vi "XYZStage-Verify position.vi"(8 "error in (no error)":errorcluster, 10 "XYZ Stage data":T1={"Command"=enum."Dequeue", "Channel"="Z", "X"=0.0, "Y"=0.0, "Z"=0.0, "Speed"=0, "Zero"=FALSE, "Use acknowledgement?"=TRUE} {"Speed" format="Speed= %.0f"; "Z" format="Z= %#_g"; "Y" format="Y= %#_g"; "X" format="X= %#_g"}, 11 "XYZ Stage Port":refnum<visa-resource-name>) -> (0 "error out":errorcluster)   [LabVIEW 2013]
uses:
  Typedefs/XYZ stage data.ctl
  Typedefs/XYZ stage states.ctl
  Typedefs/XYZ channel ring.ctl
  Typedefs/Command acknowledgment states.ctl
  User Interface/Windows/Position control window/Globals/Pos ctrl window globals.vi
  Global Variables/gl_UI Ctrl Refs.vi
  Globals/gl_XYZStage globals.vi
panel:
  out "Iterations":i32
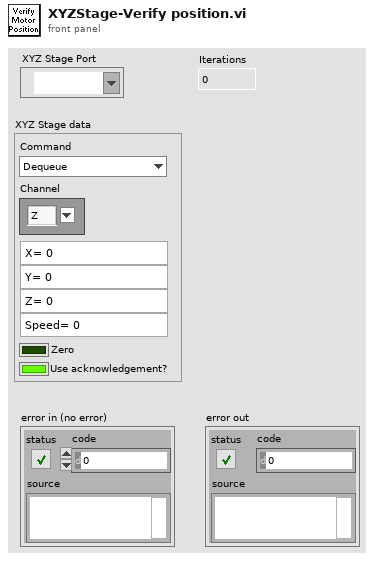
[diagram p1: front panel]
types:
  T1 = typedef "XYZ stage data.ctl" = cluster{"Command":T2, "Channel":T3, "X":sgl, "Y":sgl, "Z":sgl, "Speed":i32, "Zero":bool, "Use acknowledgement?":bool}
  T2 = typedef "XYZ stage states.ctl" = enum16{"Dequeue", "Initialize", "Read Position", "Read Speed Setting", "Move", "Set Max Speed", "Reset Axis", "Stop all movement"}
  T3 = typedef "XYZ channel ring.ctl" = string
  T4 = typedef "Command acknowledgment states.ctl" = enum16{"Acknowledge", "Wait for acknowledgment", "Release queue"}
  T5 = typedef "UI ctrl refs cluster.ctl" = cluster{"Top level VI path":path, "Top level VI ref":refnum<vi>, "User menu ref":refnum<k9>, "Sub Panel control":refnum<vi>, "Imaging Param Tab":refnum<vi>, "Occurrence-Start drivers":refnum<k4>, "Occurrence-Speed logging initialised":refnum<k4>, "Occurrence-XYZ stage initialised":refnum<k4>, "Exit button":refnum<vi>, "Status ind":refnum<vi>, "Return to Origin":refnum<vi>, "Speed Logging":refnum<vi>, "Time Lapse":refnum<vi>, "Live Imaging":refnum<vi>, "AOL Z Stack":refnum<vi>, "Motor Z Stack":refnum<vi>, "Funct Acq button":refnum<vi>, "Hard Shutter":refnum<vi>, "Virtual Shutter":refnum<vi>, "Laser Power":refnum<vi>, "AOL Mode":refnum<vi>, "Frame Size":refnum<vi>, "Field of View":refnum<vi>, "Dwell Time":refnum<vi>, "Zoom":refnum<vi>, "AOL Z":refnum<vi>, "Objective":refnum<vi>, "Axis":refnum<vi>, "Paths & Names":refnum<vi>, "Experiment folder path (ind.)":refnum<vi>, "Last State (Ind.)":refnum<vi>, "Laser wavelength ind (nm)":refnum<vi>, "Averages":refnum<vi>, "Angle (degrees)":refnum<vi>, "X centre":refnum<vi>, "Y centre":refnum<vi>, "Plane Mode":refnum<vi>, "# Planes":refnum<vi>, "Z Start":refnum<vi>, "Z Stop":refnum<vi>, "Z Step":refnum<vi>, "PMT 1":refnum<vi>, "PMT 2":refnum<vi>, "Stage XYZ Position":refnum<vi>, "Pockels@Z Start":refnum<vi>, "Pockels@Z Stop":refnum<vi>, "Obtain Z Start":refnum<vi>, "Obtain Z Stop":refnum<vi>, "Live stim.trig.period":refnum<vi>, "Live stim.trig.enable":refnum<vi>, "Funct. Acq. Pockels Modulation":refnum<vi>, "Enable Video Recording":refnum<vi>, "Video Record-Live Imaging":refnum<vi>, "Video Record-Funct acq":refnum<vi>, "AOL Z-stack Chirps Ready (ind)":refnum<vi>, "Center freq ind (nm)":refnum<vi>, "Logging queue (ind)":refnum<vi>, "Back aperture power (ind.)":refnum<vi>, "Power after objective (ind.)":refnum<vi>, "Switch user":refnum<vi>}
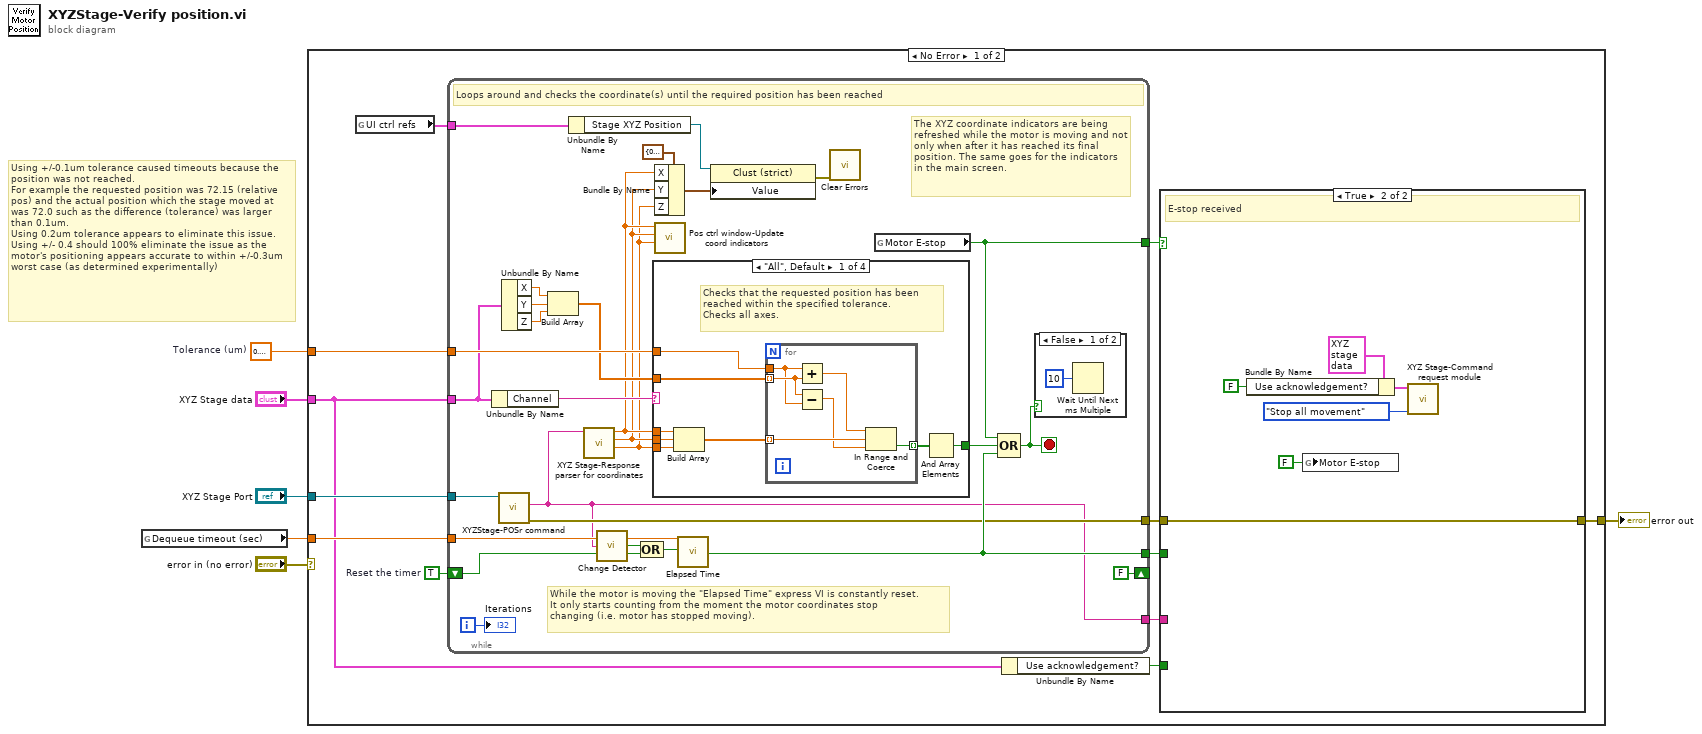
[diagram p0: block diagram]
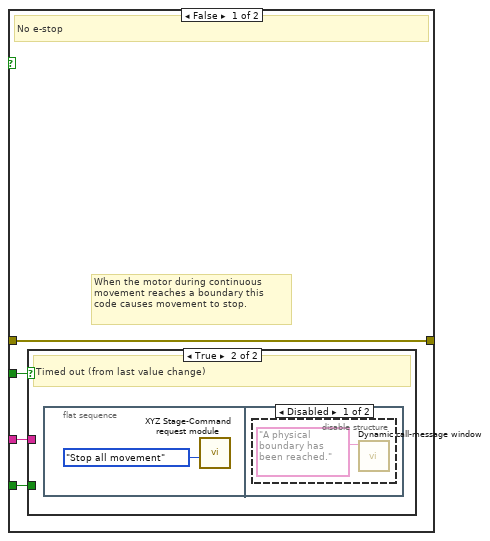
[diagram p2: hidden frame]
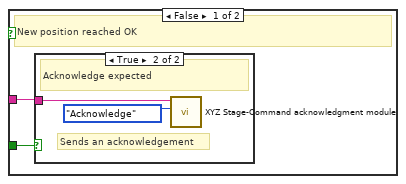
[diagram p3: hidden frame]
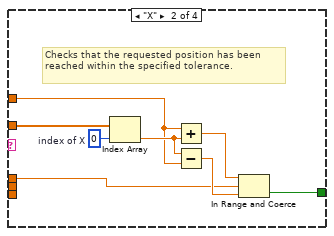
[diagram p6: hidden frame]
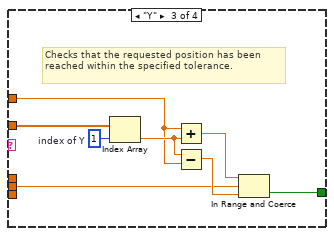
[diagram p7: hidden frame]
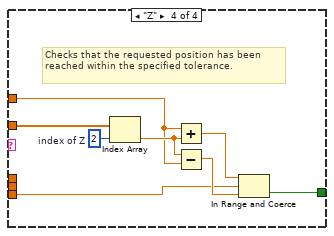
[diagram p8: hidden frame]
diagram:
  w2 = sgl 0.4  # Tolerance (um)
  # "Using +/-0.1um tolerance caused timeouts because the position was not reached.\nFor example the requested position was 72.15 (relative pos) and the actual position which the stage moved at was 72.0 such as the difference (tolerance) was larger than 0.1um.\nUsing 0.2um tolerance appears to eliminate this issue.\nUsing +/- 0.4 should 100% eliminate the issue as the motor's positioning appears accurate to within +/-0.3um worst case (as determined experimentally)"
  n1 = global read "Pos ctrl window globals.vi" "Dequeue timeout (sec)"() -> (w1:dbl)
  n2 = case shown="No Error" "error in (no error)" {
    selector: "error in (no error)" -> [_ w102]
    tunnel: "XYZ Stage data" -> [w11 _]
    tunnel: "XYZ Stage Port" -> [w18 _]
    tunnel: [w7 w102] -> w3
    tunnel: w1 -> [w16 _]
    tunnel: w2 -> [w15 _]
    frame No Error {
      w17 = TRUE  # Reset the timer
      n3 = global read "gl_UI Ctrl Refs.vi" "UI ctrl refs"() -> (w14:T5)
      n4 = while {
        tunnel: [w37] -> w8
        tunnel: w18 -> [w38]
        tunnel: w11 -> [w51]
        shift-right: [FALSE ("Send command")] -> _
        shift-left: w17 -> [w53]
        tunnel: w15 -> [w60]
        tunnel: w16 -> [w59]
        tunnel: [w56] -> w13
        tunnel: [w36] -> w12
        tunnel: w14 -> [w42]
        tunnel: [w35] -> w9
        i -> [w55]
        stop <- w58 stop-if-true
        # "The XYZ coordinate indicators are being refreshed while the motor is moving and not only when after it has reached its final position. The same goes for the indicators in the main screen."
        # "While the motor is moving the \"Elapsed Time\" express VI is constantly reset.\nIt only starts counting from the moment the motor coordinates stop \nchanging (i.e. motor has stopped moving)."
        # "Loops around and checks the coordinate(s) until the required position has been reached"
        n5 = Unbundle By Name(w51) -> ("Channel"=w61:T3)
        n6 = call "XYZStage-POSr command.vi"("VISA Refnum in"=w38) -> ("Error out"=w37:errorcluster, "read string"=w36:string)  [unwired: 7 in, 2 out]
        n7 = Unbundle By Name(w51) -> ("X"=w49:sgl, "Y"=w50:sgl, "Z"=w48:sgl)
        n8 = Build Array(w49, w50, w48) -> (w47:sgl[])
        n9 = Unbundle By Name(w42) -> ("Stage XYZ Position"=w46:refnum<vi>)
        n10 = call "XYZ Stage-Response parser for coordinates.vi"("Filtered response string (no CR)"=w36) -> ("Z"=w39:sgl, "Y"=w40:sgl, "X"=w41:sgl)  [unwired: 8 in]
        n11 = call "Change Detector.vi"("Value"=w36) -> ("Changed?"=w54:bool)
        n12 = Compound Arithmetic op=OR(w54, w53) -> (w52:bool)
        n13 = case shown="\"All\", Default" w61 {
          tunnel: w41 -> [w70 w78 _ _]
          tunnel: w40 -> [w69 _ w85 _]
          tunnel: w39 -> [w68 _ _ w93]
          tunnel: [w65 w77 w86 w94] -> w57
          tunnel: w47 -> [w64 w81 w89 w97]
          tunnel: w60 -> [w63 w79 w87 w95]
          frame "All", Default {
            # "Checks that the requested position has been reached within the specified tolerance.\nChecks all axes."
            n14 = Build Array(w70, w69, w68) -> (w67:sgl[])
            n15 = for {
              tunnel: w64 -> [w75] mode=indexing
              tunnel: w67 -> [w76] mode=indexing
              tunnel: [w72] -> w66 mode=indexing
              tunnel: w63 -> [w71]
              n16 = Add(x=w71, y=w75) -> (x+y=w74:sgl)
              n17 = Subtract(x=w75, y=w71) -> (x-y=w73:sgl)
              n18 = In Range and Coerce(upper limit=w74, x=w76, lower limit=w73) -> (In Range?=w72:bool)  [unwired: 1 out]
            }
            n19 = And Array Elements(Boolean array=w66) -> (logical AND=w65:bool)
          }
          frame "X" {
            w82 = 0  # index of X
            # "Checks that the requested position has been reached within the specified tolerance."
            n20 = Index Array(array=w81, index=w82) -> (element=w80:sgl)
            n21 = Add(x=w79, y=w80) -> (x+y=w84:sgl)
            n22 = Subtract(x=w80, y=w79) -> (x-y=w83:sgl)
            n23 = In Range and Coerce(upper limit=w84, x=w78, lower limit=w83) -> (In Range?=w77:bool)  [unwired: 1 out]
          }
          frame "Y" {
            w90 = 1  # index of Y
            # "Checks that the requested position has been reached within the specified tolerance."
            n24 = Index Array(array=w89, index=w90) -> (element=w88:sgl)
            n25 = Add(x=w87, y=w88) -> (x+y=w92:sgl)
            n26 = Subtract(x=w88, y=w87) -> (x-y=w91:sgl)
            n27 = In Range and Coerce(upper limit=w92, x=w85, lower limit=w91) -> (In Range?=w86:bool)  [unwired: 1 out]
          }
          frame "Z" {
            w98 = 2  # index of Z
            # "Checks that the requested position has been reached within the specified tolerance."
            n28 = Index Array(array=w97, index=w98) -> (element=w96:sgl)
            n29 = Add(x=w95, y=w96) -> (x+y=w100:sgl)
            n30 = Subtract(x=w96, y=w95) -> (x-y=w99:sgl)
            n31 = In Range and Coerce(upper limit=w100, x=w93, lower limit=w99) -> (In Range?=w94:bool)  [unwired: 1 out]
          }
        }
        n32 = Bundle By Name(cluster=cluster{"X":sgl, "Y":sgl, "Z":sgl} {"X"=0.0, "Y"=0.0, "Z"=0.0} ("Stage XYZ Position"), "X"=w41, "Y"=w40, "Z"=w39) -> (w44:cluster{"X":sgl, "Y":sgl, "Z":sgl})
        n33 = call "Pos ctrl window-Update coord indicators.vi"("Z"=w39, "Y"=w40, "X"=w41) -> ()  [unwired: 9 in]
        n34 = call "Elapsed Time"("Time Target (s)"=w59, "Reset"=w52) -> ("Time has Elapsed"=w56:bool)  [unwired: 10 in, 7 out]
        n35 = property on="Property Node" class="Clust (strict)"(reference=w46, "Value"=w44) -> (error out=w45:errorcluster)  [unwired: 1 in, 1 out]
        n36 = call <vilib>:"Clear Errors.vi"("error in (no error)"=w45) -> ()  [unwired: 6 in, 1 out]
        n37 = global read "gl_XYZStage globals.vi" "Motor E-stop"() -> (w35:bool)
        n38 = Compound Arithmetic op=OR(w35, w57, w56) -> (w58:bool)
        n39 = case shown="False" w58 {
          frame False {
            n40 = Wait Until Next ms Multiple(millisecond multiple=u32 10) -> ()  [unwired: 1 out]
          }
          frame True {
            # "No wait if position reached"
          }
        }
        "Iterations" <- w55
      }
      n41 = Unbundle By Name(w11) -> ("Use acknowledgement?"=w10:bool)
      n42 = case shown="True" w9 {
        tunnel: w13 -> [w22 _]
        tunnel: w12 -> [w21 _]
        tunnel: w10 -> [w20 _]
        tunnel: w8 -> [w19 w32]
        tunnel: [w19 w32] -> w7
        frame False {
          # "When the motor during continuous movement reaches a boundary this code causes movement to stop."
          # "No e-stop"
          n43 = case shown="True" w22 {
            tunnel: w21 -> [w24 _]
            tunnel: w20 -> [w23 _]
            frame False {
              # "New position reached OK"
              n44 = case shown="True" w23 {
                tunnel: w24 -> [_ w25]
                frame False {
                  # "No acknowledgement expected"
                }
                frame True {
                  # "Sends an acknowledgement"
                  # "Acknowledge expected"
                  n45 = call "XYZ Stage-Command acknowledgment module.vi"("State"=Command_acknowledgment_states."Acknowledge", "Acknowledgement Message in"=w25) -> ()  [unwired: 7 in, 3 out]
                }
              }
            }
            frame True {
              # "Timed out (from last value change)"
              n46 = flat-sequence {
                frame #0 {
                  n47 = call "XYZ Stage-Command request module.vi"("Command"=XYZ_stage_states."Stop all movement") -> ()  [unwired: 6 in, 5 out]
                }
                frame #1 {
                  n48 = disable-structure shown="Disabled" {
                    frame Disabled {
                      n49 = call "Dynamic call-message window.vi"("Message"="A physical boundary has been reached." ("Error Message")) -> ()  [unwired: 10 in, 1 out]
                    }
                    frame Enabled {
                    }
                  }
                }
              }
            }
          }
        }
        frame True {
          # "E-stop received"
          n50 = Bundle By Name(cluster=T1 {"Command"=enum."Initialize", "Channel"="Z", "X"=0.0, "Y"=0.0, "Z"=0.0, "Speed"=0, "Zero"=FALSE, "Use acknowledgement?"=TRUE} ("XYZ Stage data to queue"), "Use acknowledgement?"=FALSE) -> (w30:T1)
          n51 = global write "gl_XYZStage globals.vi" "Motor E-stop"(FALSE ("Motor E-stop")) -> ()
          n52 = call "XYZ Stage-Command request module.vi"("Command"=XYZ_stage_states."Stop all movement", "XYZ Stage data to queue"=w30) -> ()  [unwired: 5 in, 5 out]
        }
      }
    }
    frame Error {
    }
  }
  "error out" <- w3
